vi "LoadingWindow.vi"(11 "channel":T1) -> ()   [LabVIEW 2024]
uses:
  <extravilib>/ChannelInstances/Stream-str/)Channel.ctl
  <extravilib>/ChannelInstances/Tag-bool/Read With Abort.vi
  <extravilib>/ChannelInstances/Stream-str/Read With Abort.vi
  <extravilib>/ChannelInstances/Tag-bool/Write With Abort.vi
  <extravilib>/ChannelInstances/Stream-str/EndpointRead.vi
  <extravilib>/ChannelInstances/Tag-bool/Instantiate.vi
  <extravilib>/ChannelInstances/Tag-bool/EndpointRead.vi
  <extravilib>/ChannelInstances/Stream-str/)Channel.vi
  <resource>/ChannelSupport/_ChannelSupport/WaitIfNeeded.vi
  <extravilib>/ChannelInstances/Tag-bool/Endpoint.vi
  <extravilib>/ChannelInstances/Tag-bool.lvlib
  <extravilib>/ChannelInstances/Stream-str.lvlib
panel:
  out "Description_Long":string
  out "Progress":dbl(slide) scale=0.0..14.0
  out "Description":string
  out "Task":string
  out "Version":string
  # "BioSIM"
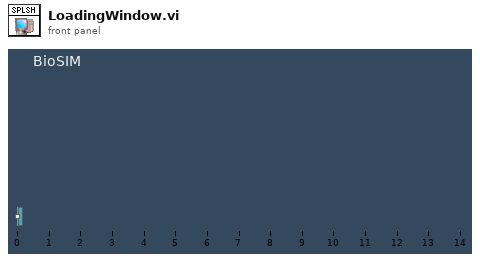
[diagram p1: front panel]
types:
  T1 = typedef "Stream-str.lvlib/)Channel.ctl" = refnum<queue>
  T2 = enum32{"Invalid", "Standard", "Closed", "Hidden", "Minimized", "Maximized"}
  T3 = enum32{"invalid app kind", "Development System", "Run Time System", "Student Edition", "Embedded LabVIEW", "Evaluation", "Custom"}
  T4 = cluster{"Core":cluster{"Current VI Reference":refnum<vi>, "Close Panel on Exit?":bool}}
  T5 = cluster{"Current VI Reference":refnum<vi>, "Close Panel on Exit?":bool}
  T6 = typedef "Tag-bool.lvlib/))Channel.ctl" = refnum<queue>
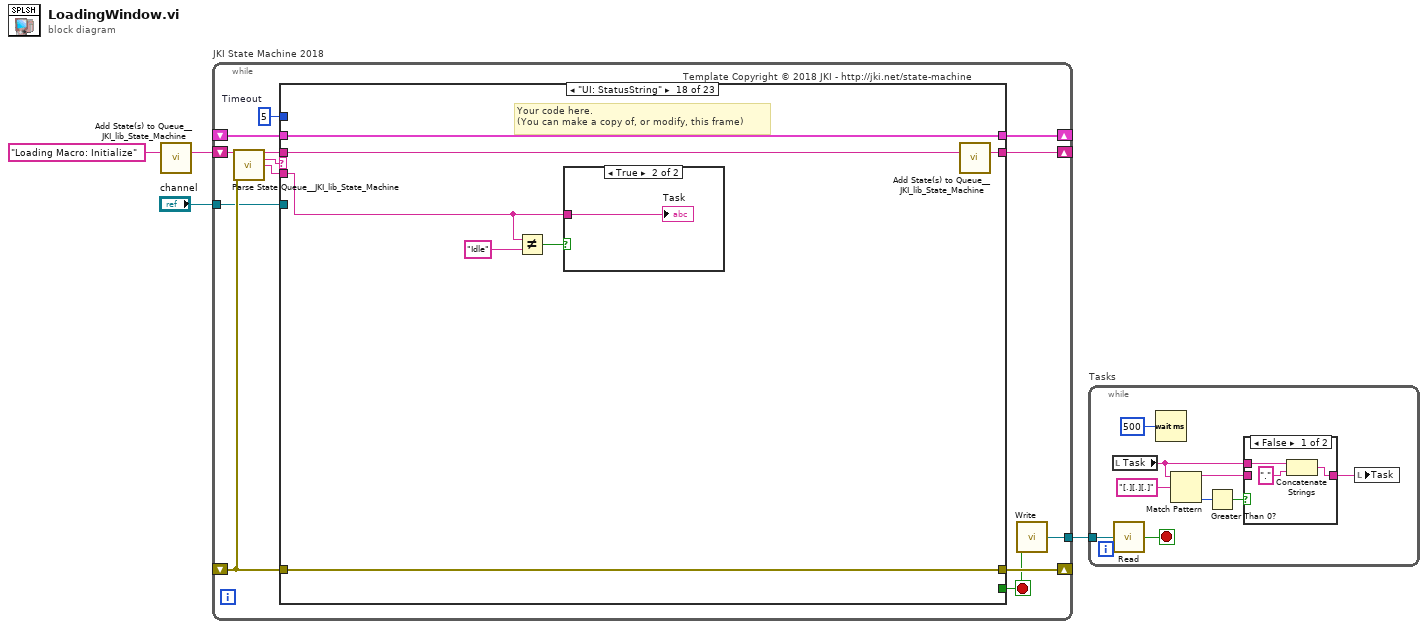
[diagram p0: block diagram]
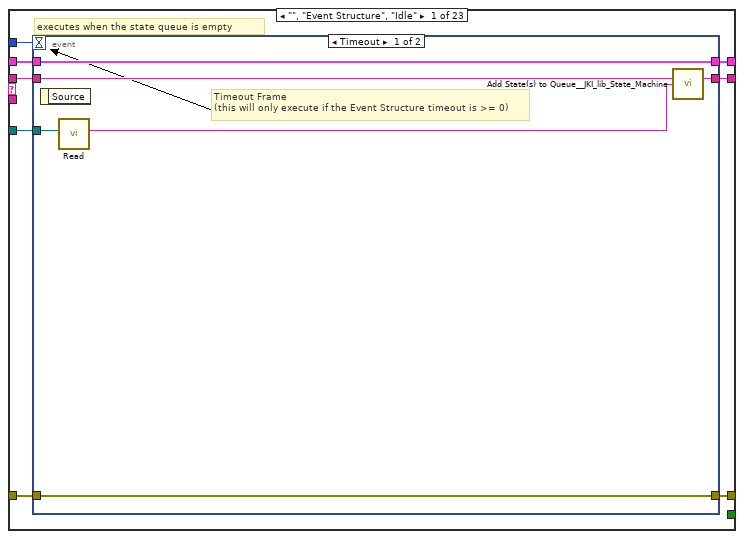
[diagram p3: hidden frame]
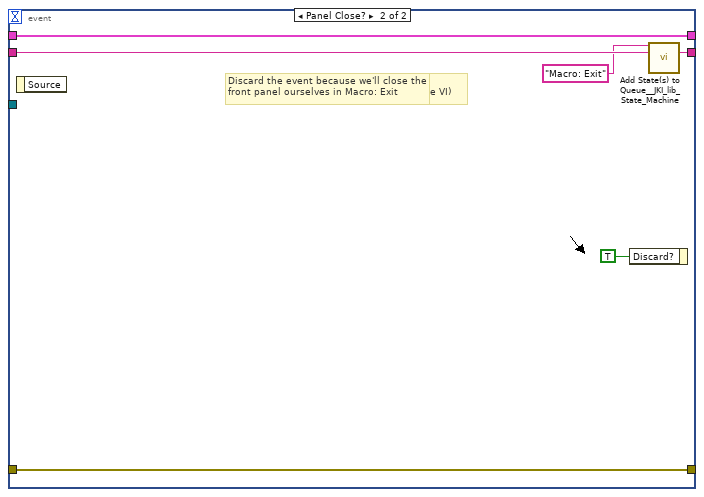
[diagram p4: hidden frame]
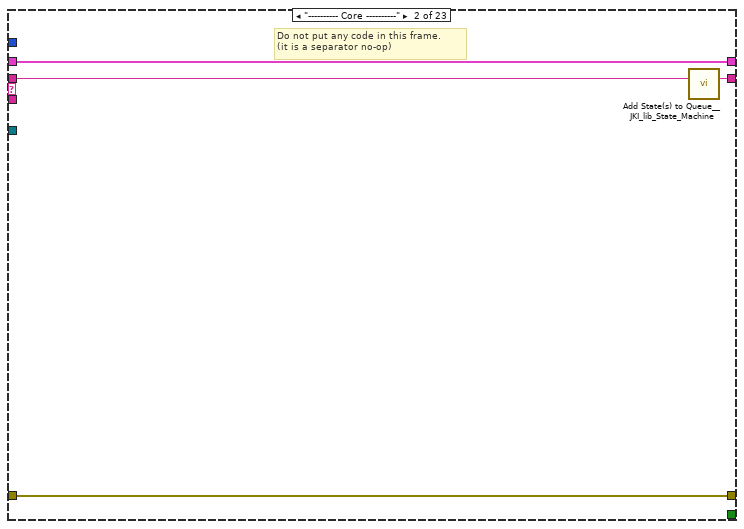
[diagram p5: hidden frame]
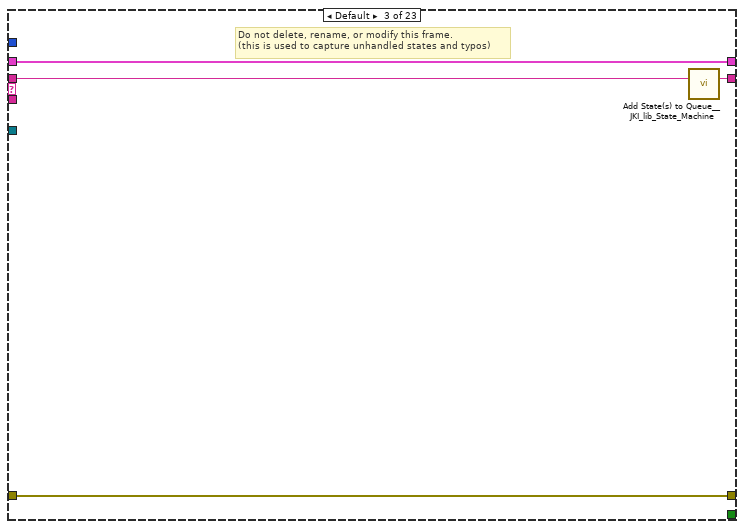
[diagram p6: hidden frame]
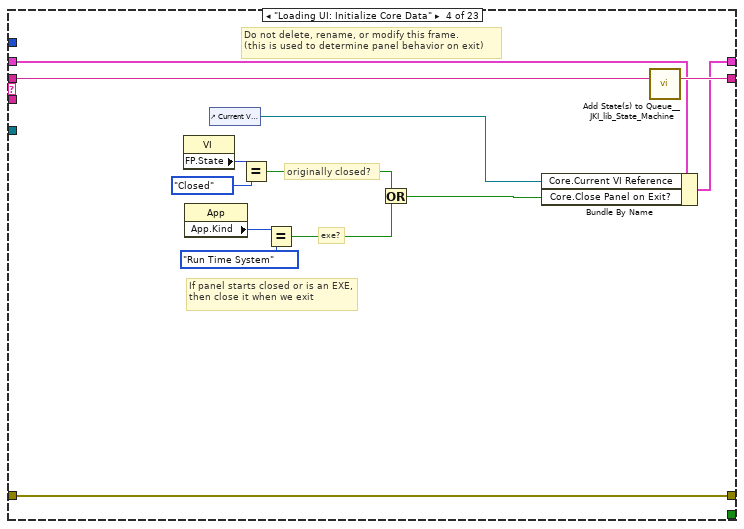
[diagram p7: hidden frame]
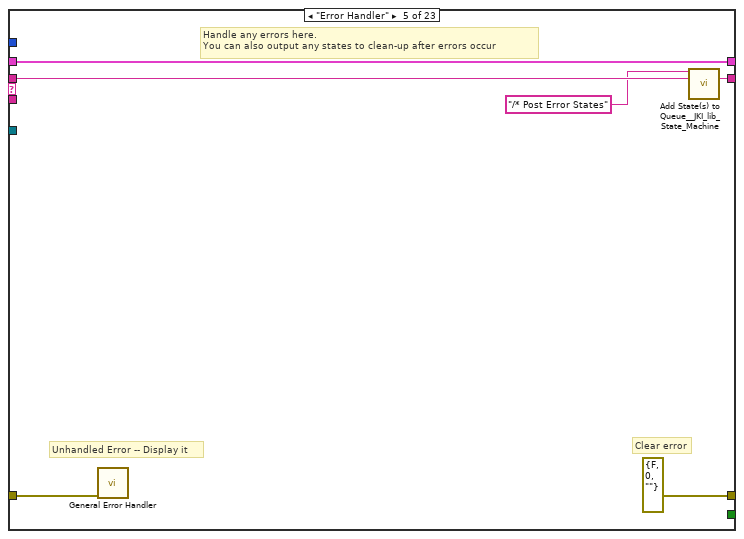
[diagram p8: hidden frame]
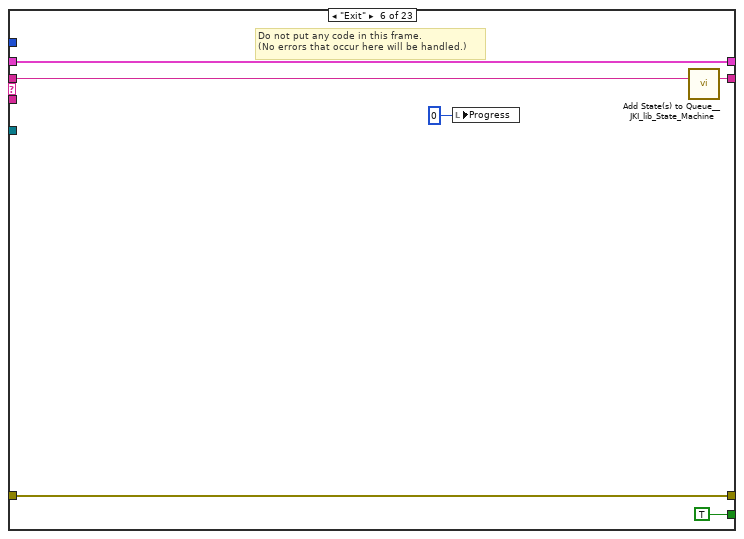
[diagram p9: hidden frame]
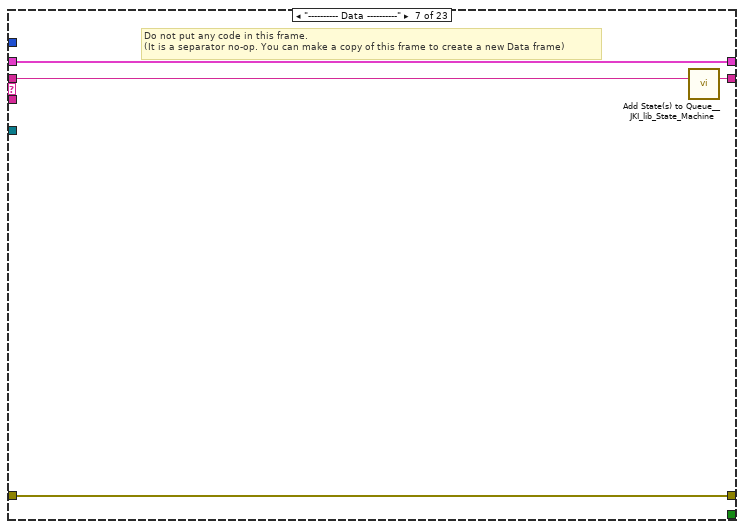
[diagram p10: hidden frame]
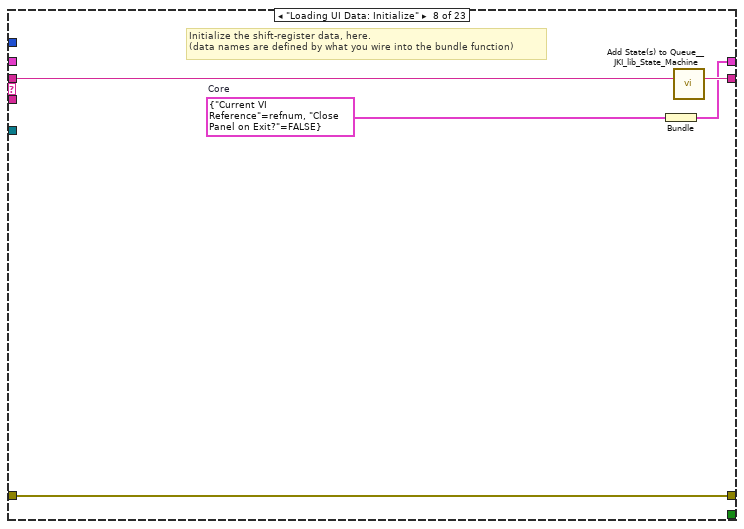
[diagram p11: hidden frame]
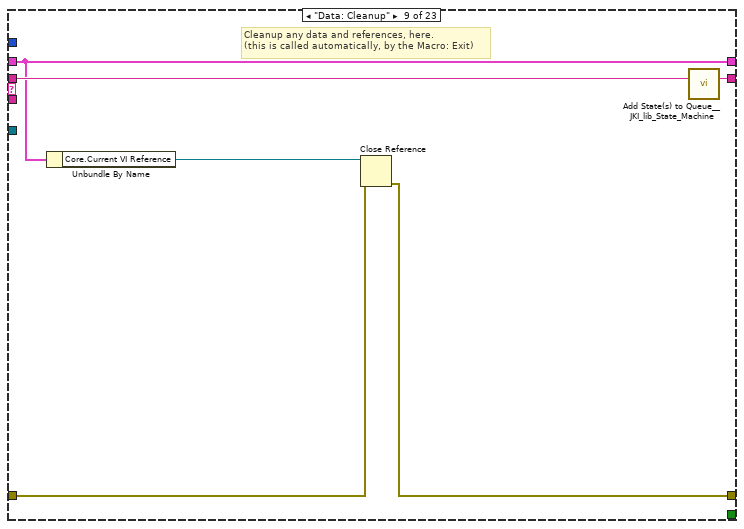
[diagram p12: hidden frame]
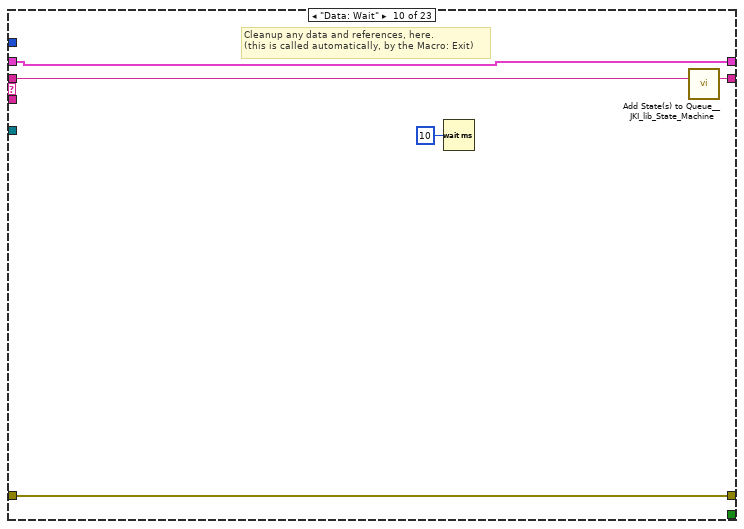
[diagram p13: hidden frame]
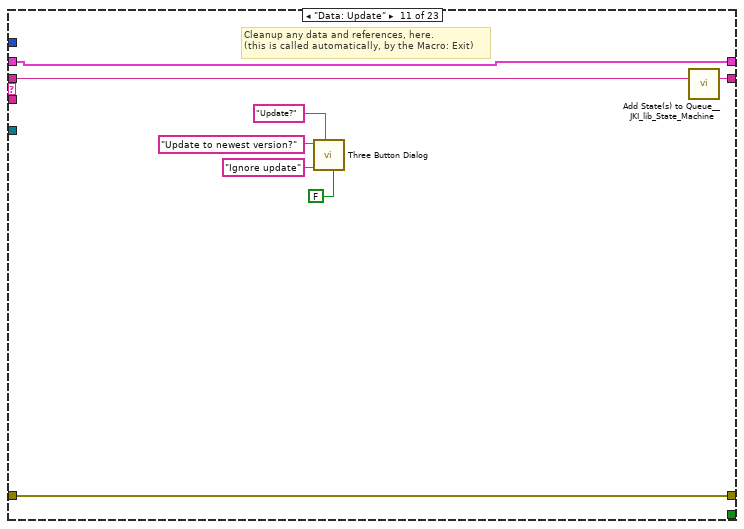
[diagram p14: hidden frame]
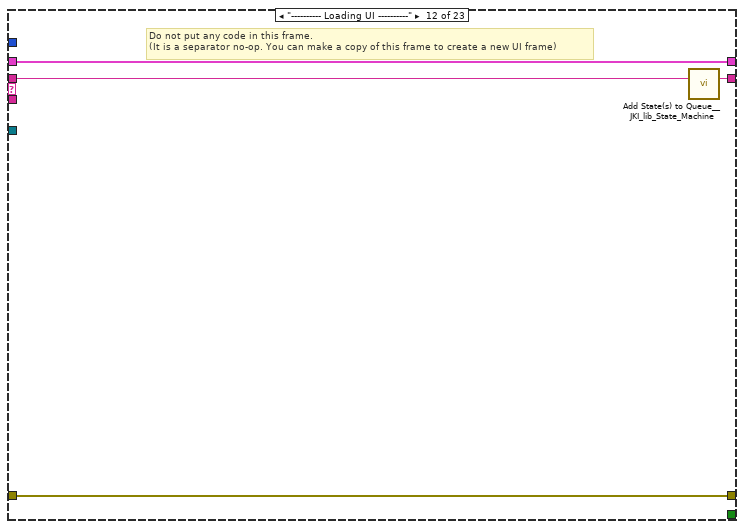
[diagram p15: hidden frame]
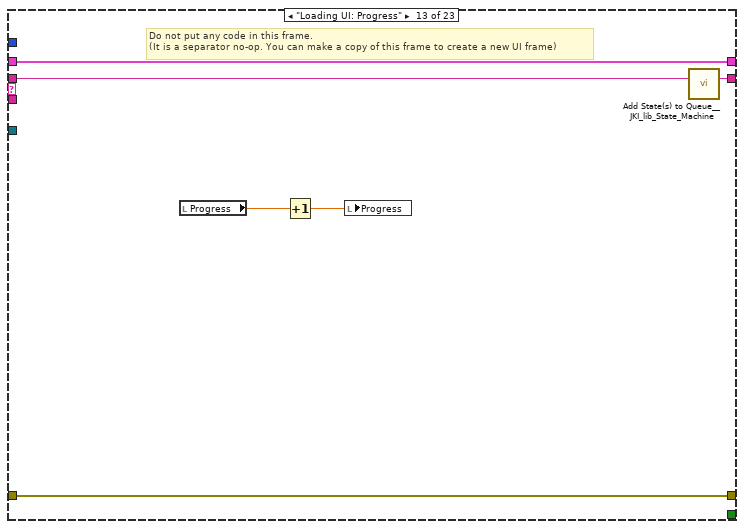
[diagram p16: hidden frame]
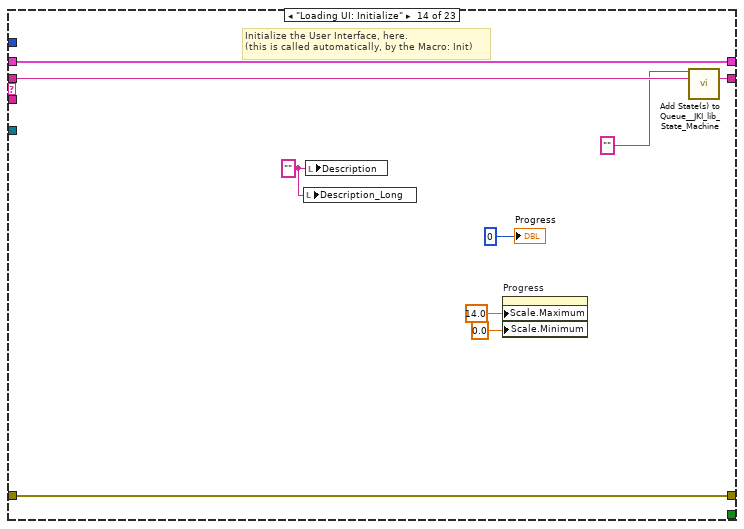
[diagram p17: hidden frame]
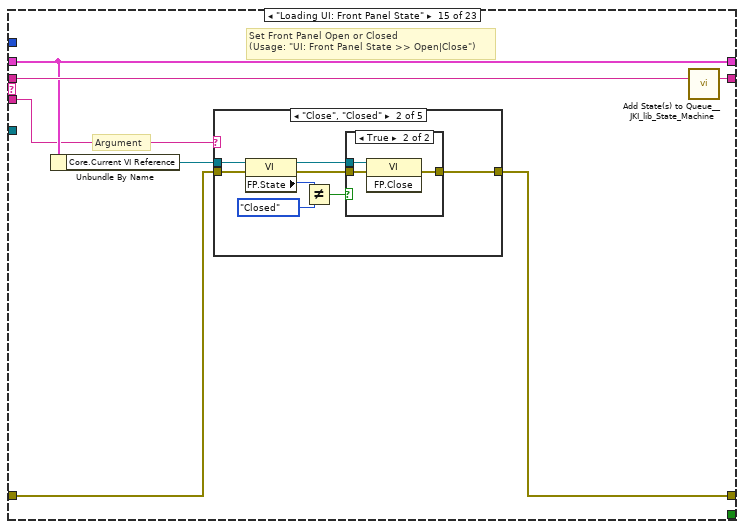
[diagram p18: hidden frame]
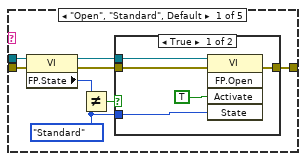
[diagram p19: hidden frame]
diagram:
  n1 = call <vilib>:"Add State(s) to Queue__JKI_lib_State_Machine.vi"("State(s) in (\"\")"="Loading Macro: Initialize") -> ("States Out"=w4:string)  [unwired: 14 in]
  n2 = while "JKI State Machine 2018" {
    shift-right: [w10] -> _
    shift-left: _ -> [w9]
    shift-right: [w13] -> _
    shift-left: _ -> [w7]
    shift-right: [w12] -> _
    shift-left: w4 -> [w14]
    tunnel: [w6] -> w1
    tunnel: "channel" -> [w5]
    stop <- w11 stop-if-true
    w8 = 5  # Timeout
    # "Template Copyright © 2018 JKI - http://jki.net/state-machine"
    n3 = call <vilib>:"Parse State Queue__JKI_lib_State_Machine.vi"("State Queue"=w14, "Error In (no error)"=w7) -> ("Remaining States"=w16:string, "Current State"=w17:string, "Arguments"=w15:string)  [unwired: 11 in]
    n4 = case shown="\"UI: StatusString\"" w17 {
      tunnel: w16 -> [w25 w41 w45 w58 w64 w70 w74 w79 w85 w90 w98 w102 w108 w117 w124 w194 w203 w211 w218 w226 w232 w238 w243]
      tunnel: w15 -> [_ _ _ _ _ _ _ _ _ _ _ _ _ _ w118 w190 w197 w206 w213 _ _ _ _]
      tunnel: w9 -> [w23 w38 w43 w51 w61 w68 w71 _ w82 w87 w95 w99 w105 w115 w120 w191 w200 w208 w216 w223 w229 w235 w240]
      tunnel: [w22 w39 w42 w55 errorcluster {"status"=FALSE, "code"=0, "source"=""} ("error out") w67 w72 w76 w80 w88 w96 w100 w106 w114 w121 w192 w201 w209 w214 w224 w230 w236 w241] -> w13
      tunnel: w7 -> [w21 w39 w42 w55 w60 w67 w72 w76 w81 w88 w96 w100 w106 w114 w122 w192 w201 w209 w215 w224 w230 w236 w241]
      tunnel: [w24 w40 w44 w57 w63 w69 w73 w78 w84 w89 w97 w101 w107 w116 w123 w193 w202 w210 w217 w225 w231 w237 w242] -> w12
      tunnel: [_ _ _ _ _ TRUE _ _ _ _ _ _ _ _ _ _ _ _ _ _ _ _ _] -> w11
      tunnel: [w20 w38 w43 w56 w61 w68 w71 w77 w82 w87 w95 w99 w105 w115 w120 w191 w200 w208 w216 w223 w229 w235 w240] -> w10
      tunnel: w8 -> [w19 _ _ _ _ _ _ _ _ _ _ _ _ _ _ _ _ _ _ _ _ _ _]
      tunnel: w5 -> [w18 _ _ _ _ _ _ _ _ _ _ _ _ _ _ _ _ _ _ _ _ _ _]
      frame "", "Event Structure", "Idle" {
        # "executes when the state queue is empty"
        n5 = event shown="[0] Timeout" {
          selector: _ -> [_ _]
          dyn-events: _ -> [_ _]
          timeout: w19 -> [_ _]
          tunnel: w25 -> [w31 w37]
          tunnel: [w30 w36] -> w24
          tunnel: w23 -> [w28 w34]
          tunnel: [w29 w35] -> w22
          tunnel: w21 -> [w29 w35]
          tunnel: [w28 w34] -> w20
          tunnel: w18 -> [w27 _]
          event Timeout {
            # "Timeout Frame\n(this will only execute if the Event Structure timeout is >= 0)"
            n6 = event-data() -> ()  [unwired: 1 in, 1 out]
            n7 = call <extravilib>:"Read.vi"("channel"=w27) -> ("element"=w26:string)  [unwired: 6 in, 4 out]
            n8 = call <vilib>:"Add State(s) to Queue__JKI_lib_State_Machine.vi"("State(s) in (\"\")"=w31, "State(s) at Back (\"\")"=w26) -> ("States Out"=w30:string)  [unwired: 13 in]
          }
          event Panel Close? {
            # "Discard the event because we'll close the front panel ourselves in Macro: Exit"
            # "Close Panel button (pressed) Event\n(this executes Macro: Exit to terminate the VI)"
            n9 = event-data() -> ()  [unwired: 1 in, 1 out]
            n10 = event-data("Discard?"=TRUE) -> ()  [unwired: 1 in, 1 out]
            n11 = call <vilib>:"Add State(s) to Queue__JKI_lib_State_Machine.vi"("State(s) in Front (\"\")"="Macro: Exit", "State(s) in (\"\")"=w37) -> ("States Out"=w36:string)  [unwired: 13 in]
          }
        }
      }
      frame "---------- Core ----------" {
        # "Do not put any code in this frame.\n(it is a separator no-op)"
        n12 = call <vilib>:"Add State(s) to Queue__JKI_lib_State_Machine.vi"("State(s) in (\"\")"=w41) -> ("States Out"=w40:string)  [unwired: 14 in]
      }
      frame Default {
        # "Do not delete, rename, or modify this frame.\n(this is used to capture unhandled states and typos)"
        n13 = call <vilib>:"Add State(s) to Queue__JKI_lib_State_Machine.vi"("State(s) in (\"\")"=w45) -> ("States Out"=w44:string)  [unwired: 14 in]
      }
      frame "Loading UI: Initialize Core Data" {
        # "Do not delete, rename, or modify this frame.\n(this is used to determine panel behavior on exit)"
        # "originally closed?"
        # "exe?"
        # "If panel starts closed or is an EXE, then close it when we exit"
        n14 = property class="VI"() -> ("FP.State"=w48:T2)  [unwired: 2 in, 2 out]
        n15 = property class="App"() -> ("App.Kind"=w54:T3)  [unwired: 2 in, 2 out]
        n16 = control-ref of="Current VI Reference"() -> (w49:refnum<vi>)
        n17 = Equal?(x=w48, y=T2."Closed" ("Front Panel Window:State")) -> (x = y?=w46:bool)
        n18 = Equal?(x=w54, y=T3."Run Time System" ("Application:Kind")) -> (x = y?=w52:bool)
        n19 = Or(x=w46, y=w52) -> (x .or. y?=w50:bool)
        n20 = Bundle By Name(cluster=w51, "Core.Current VI Reference"=w49, "Core.Close Panel on Exit?"=w50) -> (w56:T4)
        n21 = call <vilib>:"Add State(s) to Queue__JKI_lib_State_Machine.vi"("State(s) in (\"\")"=w58) -> ("States Out"=w57:string)  [unwired: 14 in]
      }
      frame "Error Handler" {
        # "Unhandled Error -- Display it"
        # "Handle any errors here.\nYou can also output any states to clean-up after errors occur"
        # "Clear error"
        n22 = call <vilib>:"General Error Handler.vi"("error in (no error)"=w60) -> ()  [unwired: 10 in, 5 out]
        n23 = call <vilib>:"Add State(s) to Queue__JKI_lib_State_Machine.vi"("State(s) in Front (\"\")"="/* Post Error States", "State(s) in (\"\")"=w64) -> ("States Out"=w63:string)  [unwired: 13 in]
      }
      frame "Exit" {
        # "Do not put any code in this frame.\n(No errors that occur here will be handled.)"
        n24 = local write "Progress"(u8 0 ("Progress")) -> ()
        n25 = call <vilib>:"Add State(s) to Queue__JKI_lib_State_Machine.vi"("State(s) in (\"\")"=w70) -> ("States Out"=w69:string)  [unwired: 14 in]
      }
      frame "---------- Data ----------" {
        # "Do not put any code in this frame.\n(It is a separator no-op. You can make a copy of this frame to create a new Data frame)"
        n26 = call <vilib>:"Add State(s) to Queue__JKI_lib_State_Machine.vi"("State(s) in (\"\")"=w74) -> ("States Out"=w73:string)  [unwired: 14 in]
      }
      frame "Loading UI Data: Initialize" {
        w75 = T5 {"Current VI Reference"=refnum, "Close Panel on Exit?"=FALSE}  # Core
        # "Initialize the shift-register data, here.\n(data names are defined by what you wire into the bundle function)"
        n27 = Bundle("Core"=w75) -> (w77:T4)  [unwired: 1 in]
        n28 = call <vilib>:"Add State(s) to Queue__JKI_lib_State_Machine.vi"("State(s) in (\"\")"=w79) -> ("States Out"=w78:string)  [unwired: 14 in]
      }
      frame "Data: Cleanup" {
        # "Cleanup any data and references, here.\n(this is called automatically, by the Macro: Exit)"
        n29 = Unbundle By Name(w82) -> ("Core.Current VI Reference"=w83:refnum<vi>)
        n30 = Close Reference(reference=w83, error in (no error)=w81) -> (error out=w80:errorcluster)
        n31 = call <vilib>:"Add State(s) to Queue__JKI_lib_State_Machine.vi"("State(s) in (\"\")"=w85) -> ("States Out"=w84:string)  [unwired: 14 in]
      }
      frame "Data: Wait" {
        # "Cleanup any data and references, here.\n(this is called automatically, by the Macro: Exit)"
        n32 = Wait (ms)(milliseconds to wait=u32 10) -> ()  [unwired: 1 out]
        n33 = call <vilib>:"Add State(s) to Queue__JKI_lib_State_Machine.vi"("State(s) in (\"\")"=w90) -> ("States Out"=w89:string)  [unwired: 14 in]
      }
      frame "Data: Update" {
        # "Cleanup any data and references, here.\n(this is called automatically, by the Macro: Exit)"
        n34 = call <vilib>:"Three Button Dialog.vi"("Allow user to close window? (TRUE)"=FALSE, "Window Title (\"\")"="Update?" ("Window Title (\"\")"), "Right Button Text (\"Cancel\")"="Ignore update" ("Right Button Text (\"Cancel\")"), "message"="Update to newest version?") -> ()  [unwired: 7 in, 1 out]
        n35 = call <vilib>:"Add State(s) to Queue__JKI_lib_State_Machine.vi"("State(s) in (\"\")"=w98) -> ("States Out"=w97:string)  [unwired: 14 in]
      }
      frame "---------- Loading UI ----------" {
        # "Do not put any code in this frame.\n(It is a separator no-op. You can make a copy of this frame to create a new UI frame)"
        n36 = call <vilib>:"Add State(s) to Queue__JKI_lib_State_Machine.vi"("State(s) in (\"\")"=w102) -> ("States Out"=w101:string)  [unwired: 14 in]
      }
      frame "Loading UI: Progress" {
        # "Do not put any code in this frame.\n(It is a separator no-op. You can make a copy of this frame to create a new UI frame)"
        n37 = local read "Progress"() -> (w104:dbl)
        n38 = Increment(x=w104) -> (x+1=w103:dbl)
        n39 = local write "Progress"(w103) -> ()
        n40 = call <vilib>:"Add State(s) to Queue__JKI_lib_State_Machine.vi"("State(s) in (\"\")"=w108) -> ("States Out"=w107:string)  [unwired: 14 in]
      }
      frame "Loading UI: Initialize" {
        w109 = "" ("Description")
        # "Initialize the User Interface, here.\n(this is called automatically, by the Macro: Init)"
        n41 = local write "Description_Long"(w109) -> ()
        n42 = local write "Description"(w109) -> ()
        n43 = property on="Progress" class="Slide (strict)"("Scale.Maximum"=14.0 ("Scale.Range:Maximum"), "Scale.Minimum"=0.0 ("Scale.Range:Minimum")) -> ()  [unwired: 2 in, 2 out]
        n44 = call <vilib>:"Add State(s) to Queue__JKI_lib_State_Machine.vi"("State(s) in Front (\"\")"="" ("State(s) in Front (\"\")"), "State(s) in (\"\")"=w117) -> ("States Out"=w116:string)  [unwired: 13 in]
        "Progress" <- u8 0 ("Progress")
      }
      frame "Loading UI: Front Panel State" {
        # "Argument"
        # "Set Front Panel Open or Closed\n(Usage: \"UI: Front Panel State >> Open|Close\")"
        n45 = Unbundle By Name(w120) -> ("Core.Current VI Reference"=w119:refnum<vi>)
        n46 = case shown="\"Close\", \"Closed\"" w118 {
          tunnel: w122 -> [w130 w145 w156 w169 w182]
          tunnel: [w132 w146 w158 w171 w184] -> w121
          tunnel: w119 -> [w131 w143 w157 w170 w183]
          frame "Open", "Standard", Default {
            w125 = T2."Standard" ("State")
            n47 = property class="VI"(reference=w131, error in=w130) -> (reference out=w128:refnum<vi>, error out=w129:errorcluster, "FP.State"=w127:T2)
            n48 = Not Equal?(x=w127, y=w125) -> (x != y?=w126:bool)
            n49 = case shown="True" w126 {
              tunnel: [w136 w138] -> w132
              tunnel: w129 -> [w135 w138]
              tunnel: w128 -> [w134 _]
              tunnel: w125 -> [w133 _]
              frame True {
                n50 = invoke class="VI" method="FP.Open"(reference=w134, error in=w135, "Activate"=TRUE, "State"=w133) -> (error out=w136:errorcluster)  [unwired: 1 in, 4 out]
              }
              frame False {
              }
            }
          }
          frame "Close", "Closed" {
            n51 = property class="VI"(reference=w143, error in=w145) -> (reference out=w142:refnum<vi>, error out=w144:errorcluster, "FP.State"=w140:T2)
            n52 = Not Equal?(x=w140, y=T2."Closed" ("Front Panel Window:State")) -> (x != y?=w139:bool)
            n53 = case shown="True" w139 {
              tunnel: [w147 w150] -> w146
              tunnel: w144 -> [w147 w149]
              tunnel: w142 -> [_ w148]
              frame False {
              }
              frame True {
                n54 = invoke class="VI" method="FP.Close"(reference=w148, error in=w149) -> (error out=w150:errorcluster)  [unwired: 1 in, 2 out]
              }
            }
          }
          frame "Hidden", "Hide" {
            w151 = T2."Hidden" ("State")
            n55 = property class="VI"(reference=w157, error in=w156) -> (reference out=w154:refnum<vi>, error out=w155:errorcluster, "FP.State"=w153:T2)
            n56 = Not Equal?(x=w153, y=w151) -> (x != y?=w152:bool)
            n57 = case shown="True" w152 {
              tunnel: [w162 w163] -> w158
              tunnel: w155 -> [w161 w163]
              tunnel: w154 -> [w160 _]
              tunnel: w151 -> [w159 _]
              frame True {
                n58 = invoke class="VI" method="FP.Open"(reference=w160, error in=w161, "State"=w159) -> (error out=w162:errorcluster)  [unwired: 2 in, 4 out]
              }
              frame False {
              }
            }
          }
          frame "Minimize", "Minimized" {
            w164 = T2."Minimized" ("State")
            n59 = property class="VI"(reference=w170, error in=w169) -> (reference out=w167:refnum<vi>, error out=w168:errorcluster, "FP.State"=w166:T2)
            n60 = Not Equal?(x=w166, y=w164) -> (x != y?=w165:bool)
            n61 = case shown="False" w165 {
              tunnel: [w175 w176] -> w171
              tunnel: w168 -> [w174 w176]
              tunnel: w167 -> [w173 _]
              tunnel: w164 -> [w172 _]
              frame True {
                n62 = invoke class="VI" method="FP.Open"(reference=w173, error in=w174, "State"=w172) -> (error out=w175:errorcluster)  [unwired: 2 in, 4 out]
              }
              frame False {
              }
            }
          }
          frame "Maximize", "Maximized" {
            w177 = T2."Maximized" ("State")
            n63 = property class="VI"(reference=w183, error in=w182) -> (reference out=w180:refnum<vi>, error out=w181:errorcluster, "FP.State"=w179:T2)
            n64 = Not Equal?(x=w179, y=w177) -> (x != y?=w178:bool)
            n65 = case shown="True" w178 {
              tunnel: [w188 w189] -> w184
              tunnel: w181 -> [w187 w189]
              tunnel: w180 -> [w186 _]
              tunnel: w177 -> [w185 _]
              frame True {
                n66 = invoke class="VI" method="FP.Open"(reference=w186, error in=w187, "State"=w185) -> (error out=w188:errorcluster)  [unwired: 2 in, 4 out]
              }
              frame False {
              }
            }
          }
        }
        n67 = call <vilib>:"Add State(s) to Queue__JKI_lib_State_Machine.vi"("State(s) in (\"\")"=w124) -> ("States Out"=w123:string)  [unwired: 14 in]
      }
      frame "Loading UI: Version" {
        # "Your code here.\n(You can make a copy of, or modify, this frame)"
        n68 = call <vilib>:"Add State(s) to Queue__JKI_lib_State_Machine.vi"("State(s) in (\"\")"=w194) -> ("States Out"=w193:string)  [unwired: 14 in]
        "Version" <- w190
      }
      frame "Loading UI: Description" {
        # "Your code here.\n(You can make a copy of, or modify, this frame)"
        n69 = local read "Description_Long"() -> (w195:string)
        n70 = case shown="\"Connections Successful\"" w197 {
          frame "False", Default {
          }
          frame "Connections Successful" {
            n71 = property on="Description" class="Str"("Text.TextColor"=u32 16448250 ("Text.Text Colors:Text Color")) -> ()  [unwired: 2 in, 2 out]
          }
        }
        n72 = Concatenate Strings(w195, w197) -> (w199:string)
        "Description" <- w199
        n73 = Concatenate Strings(w199, "\r\n") -> (→"Description_Long":string)
        n74 = call <vilib>:"Add State(s) to Queue__JKI_lib_State_Machine.vi"("State(s) in (\"\")"=w203) -> ("States Out"=w202:string)  [unwired: 14 in]
      }
      frame "UI: StatusString" {
        # "Your code here.\n(You can make a copy of, or modify, this frame)"
        n75 = Not Equal?(x=w206, y="Idle") -> (x != y?=w205:bool)
        n76 = case shown="True" w205 {
          tunnel: w206 -> [_ w212]
          frame False {
          }
          frame True {
            "Task" <- w212
          }
        }
        n77 = call <vilib>:"Add State(s) to Queue__JKI_lib_State_Machine.vi"("State(s) in (\"\")"=w211) -> ("States Out"=w210:string)  [unwired: 14 in]
      }
      frame "UI: Cursor Set" {
        # "Argument"
        # "Set and Unset Cursor Busy.\n(Usage: \"UI: Cursor Set >> Busy|Idle\")"
        n78 = case shown="\"Idle\", Default" w213 {
          tunnel: w215 -> [w220 w222]
          tunnel: [w219 w221] -> w214
          frame "Idle", Default {
            n79 = call <vilib>:"Unset Busy.vi"("error in (no error)"=w220) -> ("error out"=w219:errorcluster)  [unwired: 10 in]
          }
          frame "Busy" {
            n80 = call <vilib>:"Set Busy.vi"("error in (no error)"=w222) -> ("error out"=w221:errorcluster)  [unwired: 9 in, 1 out]
          }
        }
        n81 = call <vilib>:"Add State(s) to Queue__JKI_lib_State_Machine.vi"("State(s) in (\"\")"=w218) -> ("States Out"=w217:string)  [unwired: 14 in]
      }
      frame "---------- Macro ----------" {
        # "Do not put any code in this frame.\n(It is a separator no-op. You can make a copy of this frame to create a new Macro frame)"
        n82 = call <vilib>:"Add State(s) to Queue__JKI_lib_State_Machine.vi"("State(s) in (\"\")"=w226) -> ("States Out"=w225:string)  [unwired: 14 in]
      }
      frame "Loading Macro: Initialize" {
        # "Initialization Macro\n(This is called once, when the VI starts)"
        n83 = property on="Description" class="Str"("Text.TextColor"=u32 16711680 ("Text.Text Colors:Text Color")) -> ()  [unwired: 2 in, 2 out]
        n84 = call <vilib>:"Add State(s) to Queue__JKI_lib_State_Machine.vi"("State(s) in Front (\"\")"="Loading UI Data: Initialize\nLoading UI: Initialize Core Data\nLoading UI: Initialize\nLoading UI: Front Panel State >> Open", "State(s) in (\"\")"=w232) -> ("States Out"=w231:string)  [unwired: 13 in]
      }
      frame "Loading UI: Exit" {
        # "Exit Macro\n(This is called once, when the VI exits)"
        n85 = Wait (ms)(milliseconds to wait=u32 1500) -> ()  [unwired: 1 out]
        n86 = call <vilib>:"Add State(s) to Queue__JKI_lib_State_Machine.vi"("State(s) in Front (\"\")"="Loading UI: Front Panel State >> Close", "State(s) in (\"\")"=w238) -> ("States Out"=w237:string)  [unwired: 13 in]
      }
      frame "Macro: Exit" {
        # "Exit Macro\n(This is called once, when the VI exits)"
        n87 = call <vilib>:"Add State(s) to Queue__JKI_lib_State_Machine.vi"("State(s) in Front (\"\")"="Loading UI: Front Panel State >> Close\nExit", "State(s) in (\"\")"=w243) -> ("States Out"=w242:string)  [unwired: 13 in]
      }
    }
    n88 = call <extravilib>:"Write.vi"("element"=w11) -> ("channel"=w6:T6)  [unwired: 1 out]
  }
  n89 = while "Tasks" {
    tunnel: w1 -> [w252]
    stop <- w251 stop-if-true
    n90 = local read "Task"() -> (w246:string)
    n91 = call <extravilib>:"Read.vi"("channel"=w252) -> ("element"=w251:bool)  [unwired: 1 in, 1 out]
    n92 = Wait (ms)(milliseconds to wait=u32 500) -> ()  [unwired: 1 out]
    n93 = Match Pattern(string=w246, regular expression="[.][.][.]") -> (before substring=w248:string, offset past match=w247:i32)  [unwired: 1 in, 2 out]
    n94 = Greater Than 0?(x=w247) -> (x > 0?=w244:bool)
    n95 = case shown="False" w244 {
      tunnel: [w255 w256] -> w245
      tunnel: w246 -> [w253 _]
      tunnel: w248 -> [_ w256]
      frame False {
        n96 = Concatenate Strings(w253, "." ("string")) -> (w255:string)
      }
      frame True {
      }
    }
    n97 = local write "Task"(w245) -> ()
  }
